vi "StripDataFromVAttributes.vi"(6 "to lowercase?(F)":bool, 8 "error in (no error)":errorcluster, 11 "Map":variant) -> (0 "error out":errorcluster, 3 "duplicate variant":variant)   [LabVIEW 2019]
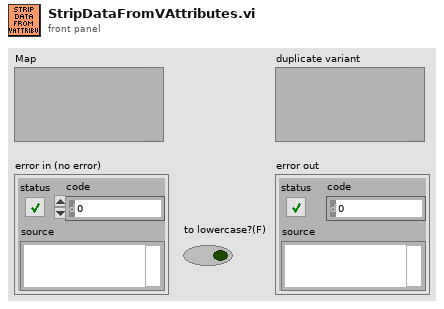
[diagram p1: front panel]
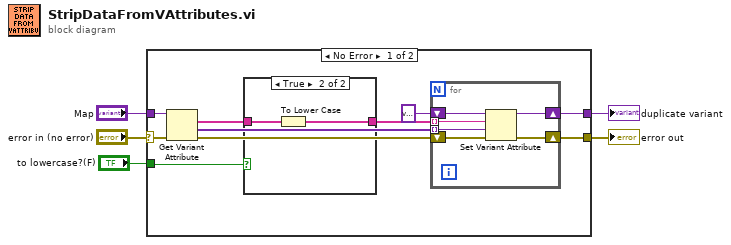
[diagram p0: block diagram]
diagram:
  n1 = case shown="No Error" "error in (no error)" {
    selector: "error in (no error)" -> [w15 w25]
    tunnel: [w13 w25] -> w4
    tunnel: [w12 _] -> w3
    tunnel: "Map" -> [w8 _]
    tunnel: "to lowercase?(F)" -> [w6 _]
    frame No Error {
      n2 = Get Variant Attribute(Variant=w8, error in=w15) -> (names=w10:string[], values=w11:variant[], error out=w14:errorcluster)  [unwired: 2 in, 1 out]
      n3 = case shown="True" w6 {
        tunnel: w10 -> [w16 w18]
        tunnel: [w16 w17] -> w7
        frame False {
        }
        frame True {
          n4 = To Lower Case(string=w18) -> (all lower case string=w17:string[])
        }
      }
      n5 = for {
        shift-right: [w23] -> w12
        shift-left: variant ("duplicate variant") -> [w24]
        tunnel: w7 -> [w22] mode=indexing
        tunnel: w11 -> [w21] mode=indexing
        shift-right: [w20] -> w13
        shift-left: w14 -> [w19]
        n6 = Set Variant Attribute(Variant=w24, name=w22, value=w21, error in=w19) -> (Variant out=w23:variant, error out=w20:errorcluster)  [unwired: 1 out]
      }
    }
    frame Error {
    }
  }
  "error out" <- w4
  "duplicate variant" <- w3
